vi "main.vi"() -> ()   [LabVIEW 2016]
uses:
  Classes/Controller/Motion/A3200 Folder/A3200.lvclass
  D:/Gantry_General/Classes/Controller/Motion/Motion Folder/Motion.lvclass
  Classes/Controller/I-O/NI-DAQ Folder/NI-DAQ.lvclass
  Classes/Controller/Dispenser/Ultimus V2 Folder/Ultimus V2.lvclass
  Classes/Controller/Motion/Motion Folder/Motion.lvclass
panel:
  in  "go patten":bool
  in  "tool go":bool
  in  "Tab Control":T1(tab)=enum."motion"
  in  "motion":T2={"XYZU "=[], "XY speed"=18.0, "Z speed"=3.0, "U speed"=0.0}
  in  "XY go":bool
  in  "Z move to zero":bool
  out "gule distances":dbl[](array[numeric])=[-11.318999999999999]
  out "needle XYZTheta In":dbl[](array[numeric])=[725.0, 1030.0, 65.0, 0.0]
  in  "needle xy":dbl[](array[numeric])=[725.0, 1030.0]
  in  "move to needle position":bool
  in  "XY":dbl[](array[numeric])=[650.0, 1030.0]
  in  "Z Go":bool
  in  "Position":dbl=65.0 format="%#_13g"
  out "j sum":dbl[](array[numeric])=[942.6350010227258, 1089.1437265164827, 59.912692205840095, 6.588294085890035e-07]
  in  "joystick and camera":bool
  in  "Camera to assembly center":bool
  out "Camera sensor center":dbl[](array[numeric])=[1019.0492232692902, 801.895067350325]
  in  "Camera to sensor center":bool
  out "sensor angle":dbl=0.7658874276042356
  in  "get sensor center":bool
  in  "get assembly center":bool
  out "Syringe offset":dbl[](array[numeric])=[-219.26459939197957, -70.034558660843, 5.209704694303774, -1.287105754835295e-06]
  out "Camera assembly center":dbl[](array[numeric])=[988.450879710852, 1092.9842118849685]
  in  "Syringe to assembly center":bool
  out "Syringe CAD center":dbl[](array[numeric])=[769.1862803188724, 1022.9496532241255]
  out "assembly angle":dbl=0.807055390089498
  in  "get Syringe offset":bool
  in  "dispense":T3={"Vacuum Setting (0000)"=200, "Pressure"=30, "on delay (ms)"=300.0, "off delay (ms) "=600.0} {"Vacuum Setting (0000)" min=0 max=1000 step=1 format="%04.0f"}
  in  "new/data":bool
  in  "dispense change status":bool
  in  "IO":cluster{"Output num":dbl[], "Output ":bool[]}={"Output num"=[11.0], "Output "=[FALSE]}
  in  "IO on /off":bool
  in  "Indices":i32[](array[numeric])=[11]
  in  "Values":bool[](array[boolean])=[TRUE]
  out "subarray":bool[](array[boolean])
  in  "z offset":T4={"Syringe Z0"=65.0, "assembly thickness"=1.219, "tool height"=9.5, "Gule thickness "=0.1, "Pick Up Tool Z height"=63.0289, "assembly Z offset"=-4.86, "gule distances"=0.6, "Syringe Z height abs"=53.681, "assembly Z height abs"=56.6499, "Syringe Z height rel"=-11.318999999999999, "assembly Z height rel"=-1.5190000000000001, "component  thickness"=0.2}
  in  "file path (dialog if empty)":path=path "D:/Gantry_General/Main/ms_kao/data/CAD patten/CAD PCB full 0.8 P30 20210608/CAD PCB full 0.8 P30 20210608.txt"
  in  "stop":bool
  in  "go CAD":bool
  in  "XY new Speed":dbl=25.0
  # "點膠速度"
  # "設定新速度"
  # "使用新/資料速度"
  # "間距70 mm"
  # "(1050, 865)\n(1050, 935)\n(1050,1005)"
  # "(910, 865)\n(910, 935)\n(910,1005)"
  # "(980, 865)\n(980, 935)\n(980,1005)"
  # "(840, 865)\n(840, 935)\n(840,1005)"
  # "0.6"
  # "PCB 1.2"
  # "sensor 0.32 ,0.2 ,0.1 mm"
  # "9.5mm"
  # "PCB 1.21"
  # "Gule 0.1mm"
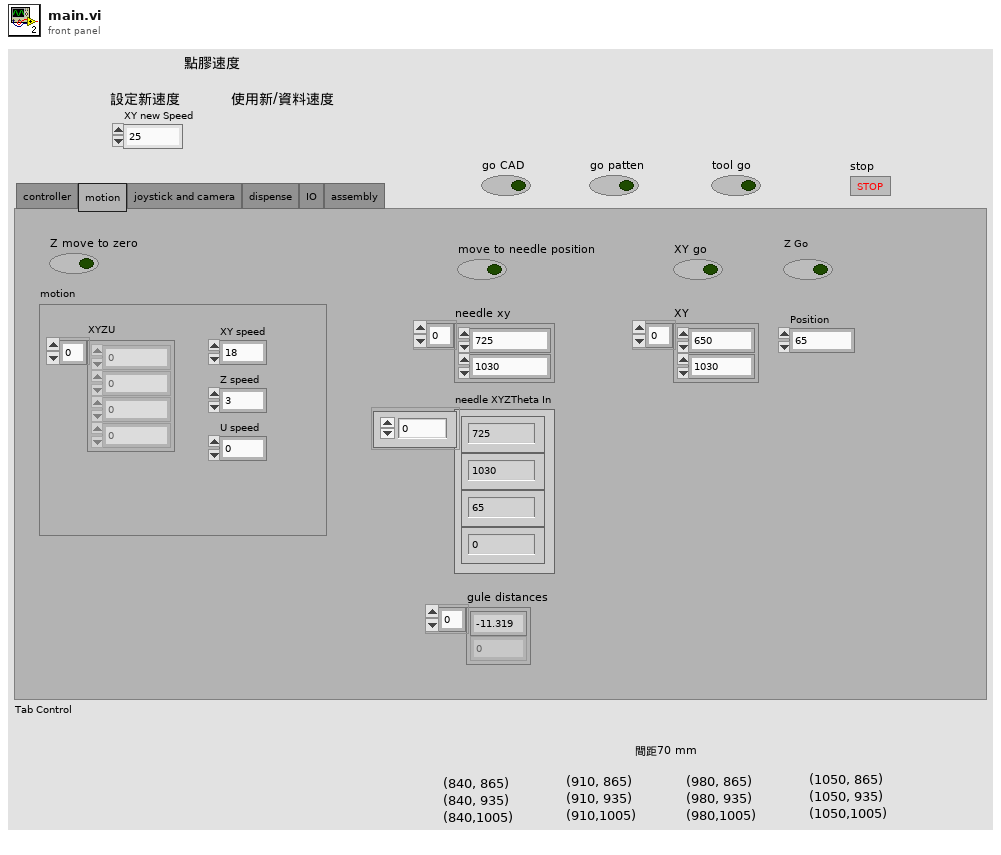
[diagram p1: front panel]
types:
  T1 = enum32{"controller", "motion", "joystick and camera", "dispense", "IO", "assembly"}
  T2 = cluster{"XYZU ":dbl[], "XY speed":dbl, "Z speed":dbl, "U speed":dbl}
  T3 = cluster{"Vacuum Setting (0000)":i64, "Pressure":i16, "on delay (ms)":dbl, "off delay (ms) ":dbl}
  T4 = cluster{"Syringe Z0":dbl, "assembly thickness":dbl, "tool height":dbl, "Gule thickness ":dbl, "Pick Up Tool Z height":dbl, "assembly Z offset":dbl, "gule distances":dbl, "Syringe Z height abs":dbl, "assembly Z height abs":dbl, "Syringe Z height rel":dbl, "assembly Z height rel":dbl, "component  thickness":dbl}
  T5 = cluster{"controller":cluster{"A3200.lvclass":refnum<class "A3200.lvclass">, "Ultimus V2.lvclass":refnum<class "Ultimus V2.lvclass">, "NI-DAQ.lvclass":refnum<class "NI-DAQ.lvclass">, "Motion.lvclass":refnum<class "Motion.lvclass">, "I-O.lvclass":refnum<class "I-O.lvclass">, "Dispenser.lvclass":refnum<class "Dispenser.lvclass">}, "folder and file name":cluster{"Path":path, "folder name":string, "file name":string, "extension":string, "add time string":bool}, "IO":cluster{"Output num":dbl[], "Output ":bool[]}, "motion":cluster{"XYZU ":dbl[], "XY speed":dbl, "Z speed":dbl, "U speed":dbl}, "dispense":cluster{"Vacuum Setting (0000)":i64, "Pressure":i16, "on delay (ms)":dbl, "off delay (ms) ":dbl}, "draw point Cluster":cluster{"dispense":bool, "Line/circle":bool, "ccw/cw":bool, "pressure":dbl, "speed":dbl, "start":dbl[], "end":dbl[], "center":dbl[], "Vacuum":dbl}}
  T6 = cluster{"A3200.lvclass":refnum<class "A3200.lvclass">, "Ultimus V2.lvclass":refnum<class "Ultimus V2.lvclass">, "NI-DAQ.lvclass":refnum<class "NI-DAQ.lvclass">, "Motion.lvclass":refnum<class "Motion.lvclass">, "I-O.lvclass":refnum<class "I-O.lvclass">, "Dispenser.lvclass":refnum<class "Dispenser.lvclass">}
  T7 = cluster{"Syringe offset":dbl[], "Camera assembly center":dbl[], "assembly angle":dbl, "Syringe CAD center":dbl[], "Camera sensor center":dbl[], "sensor angle":dbl}
  T8 = cluster{"dispense":bool, "Line/circle":bool, "ccw/cw":bool, "pressure":dbl, "speed":dbl, "start":dbl[], "end":dbl[], "center":dbl[], "Vacuum":dbl}[]
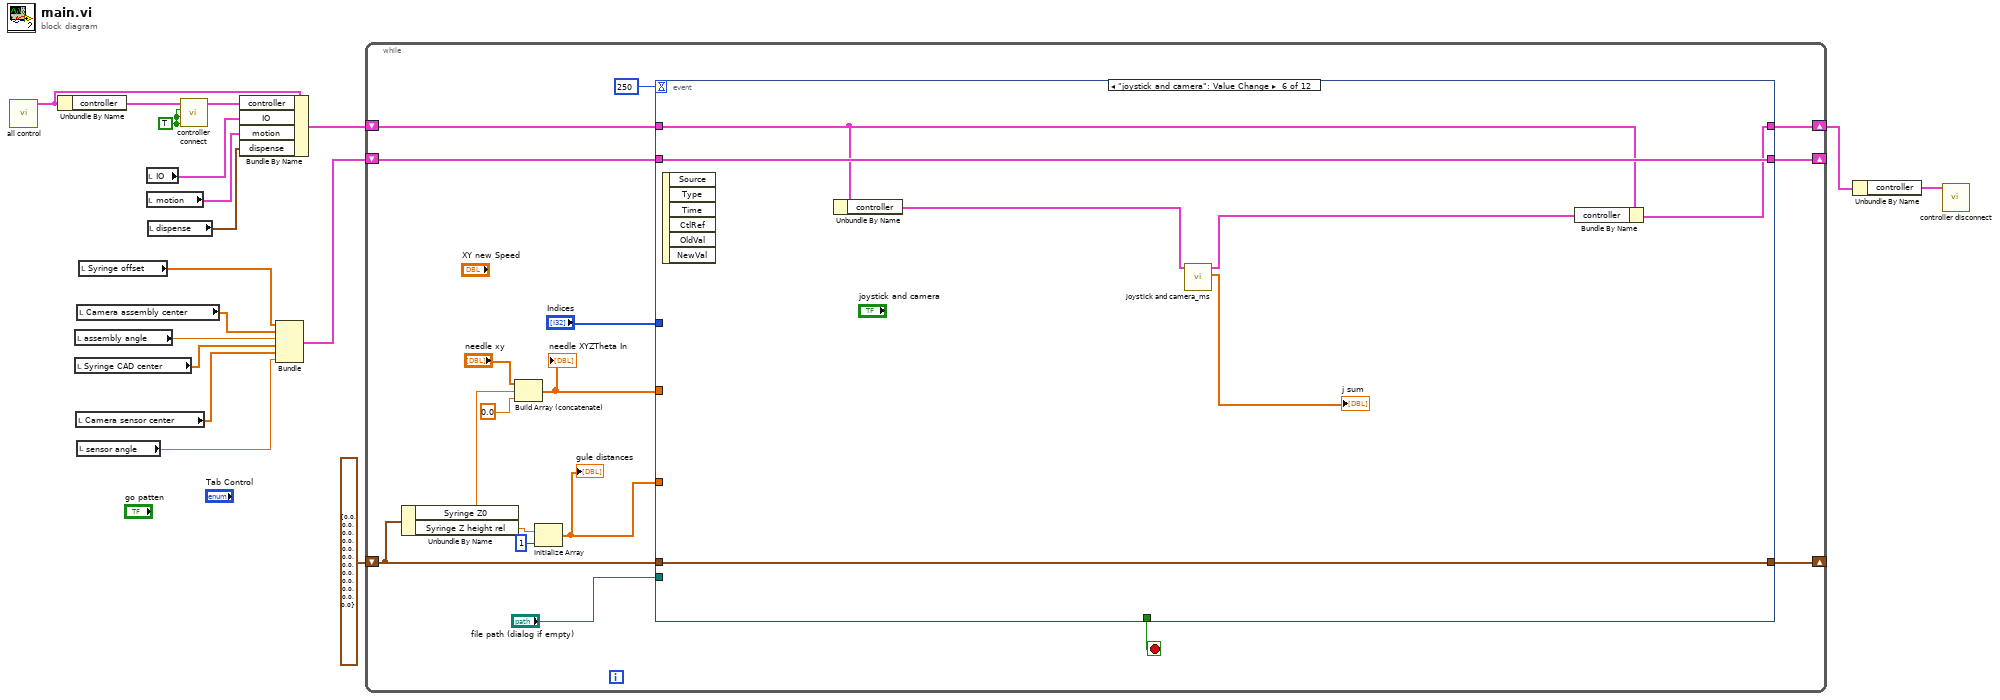
[diagram p0: block diagram]
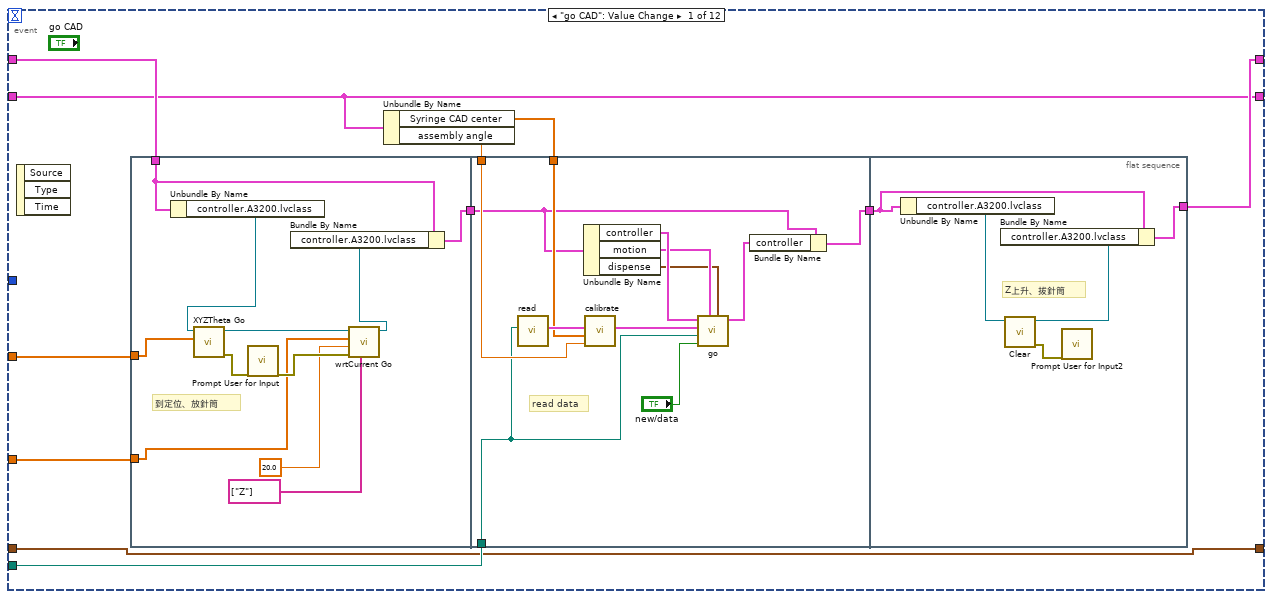
[diagram p2: hidden frame]
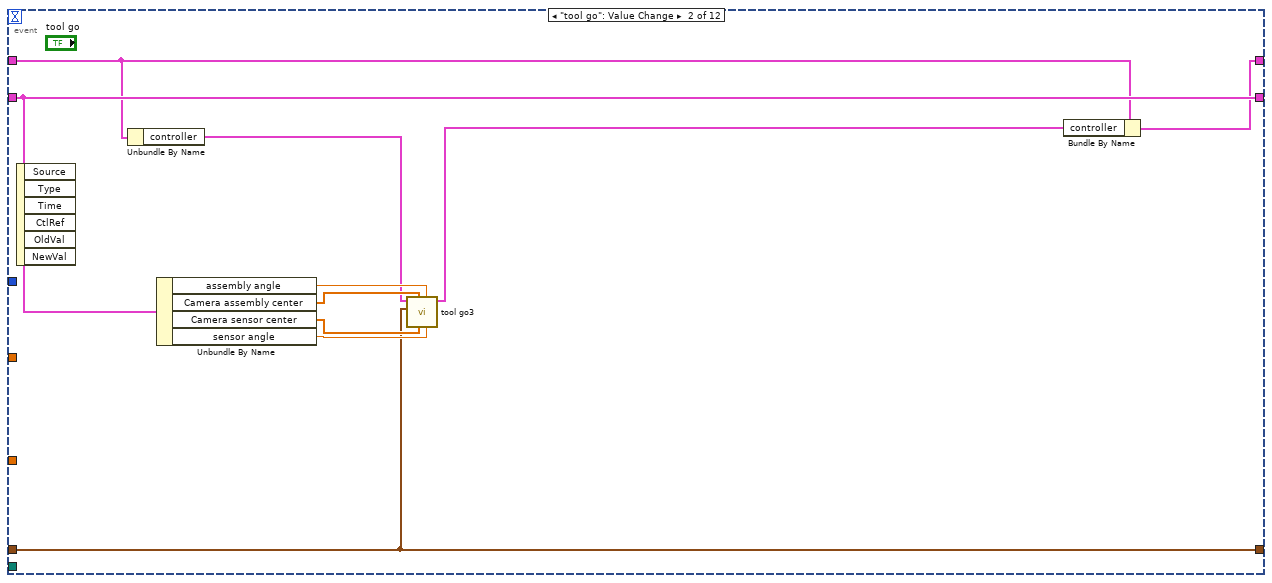
[diagram p3: hidden frame]
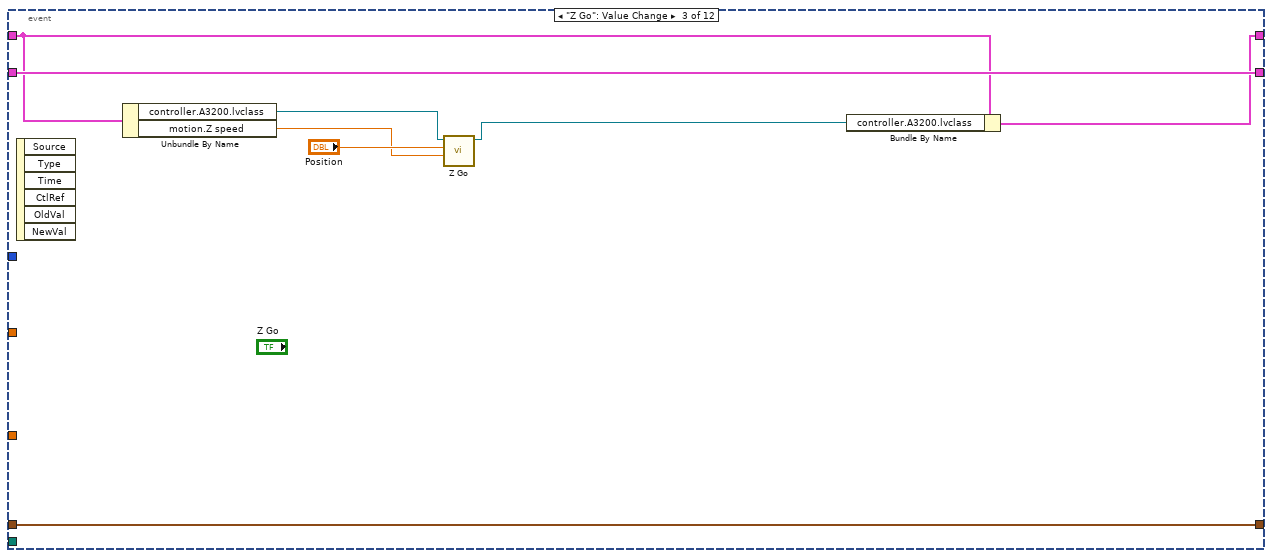
[diagram p4: hidden frame]
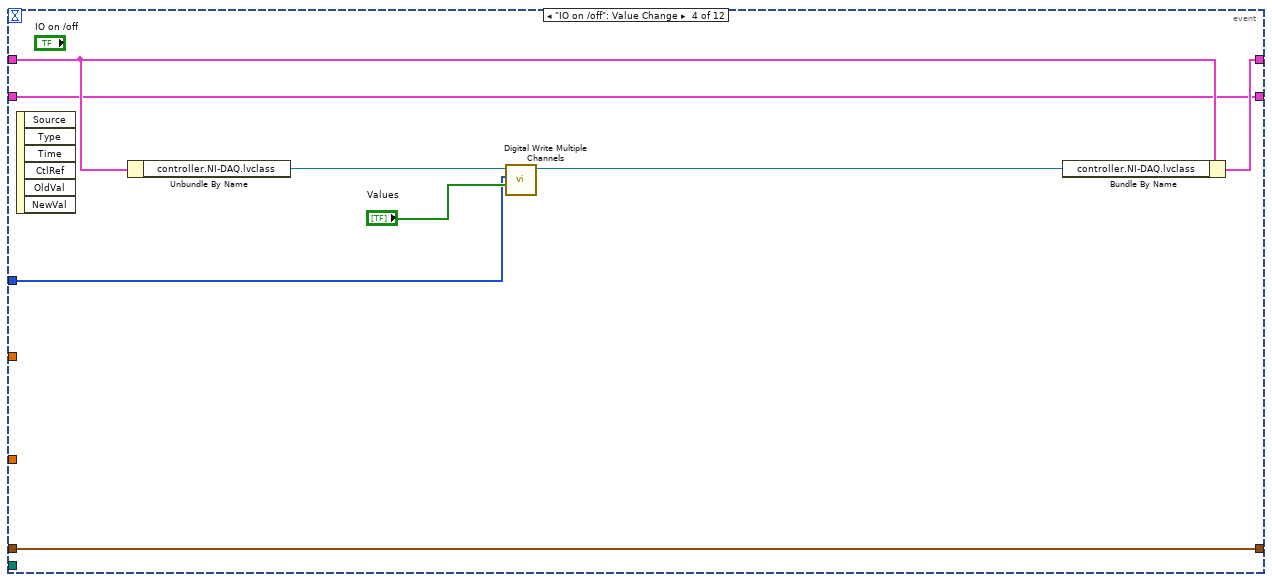
[diagram p5: hidden frame]
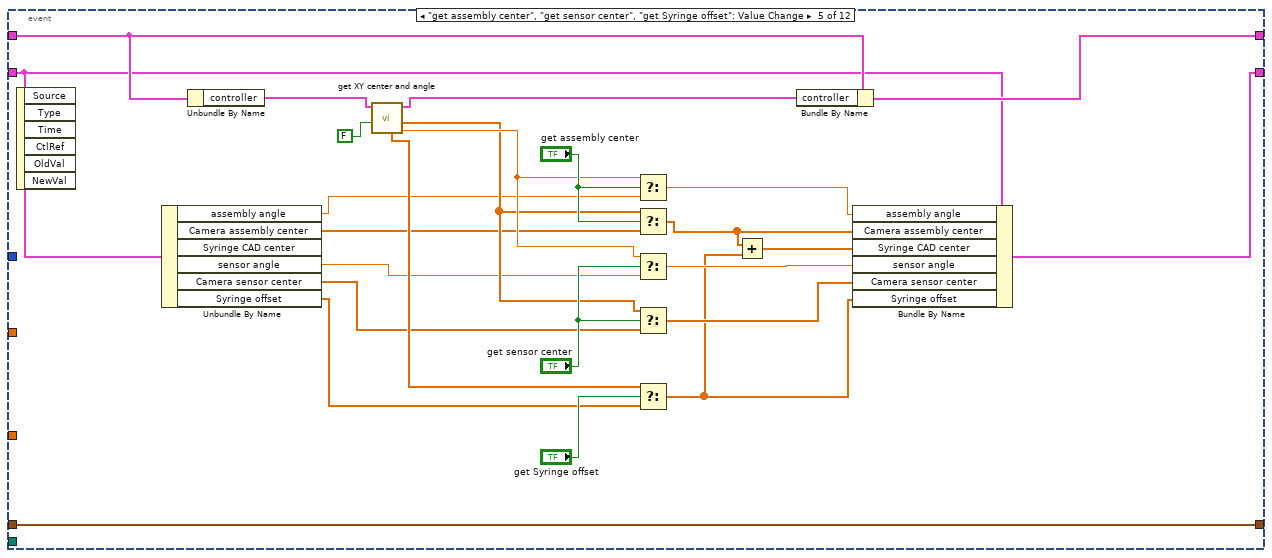
[diagram p6: hidden frame]
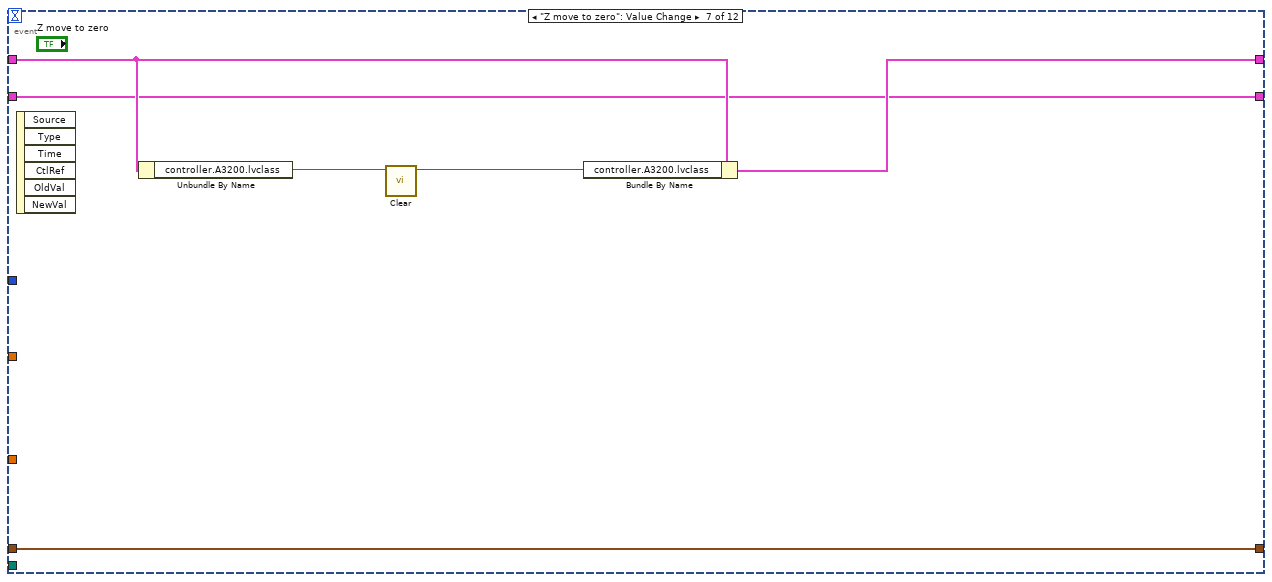
[diagram p7: hidden frame]
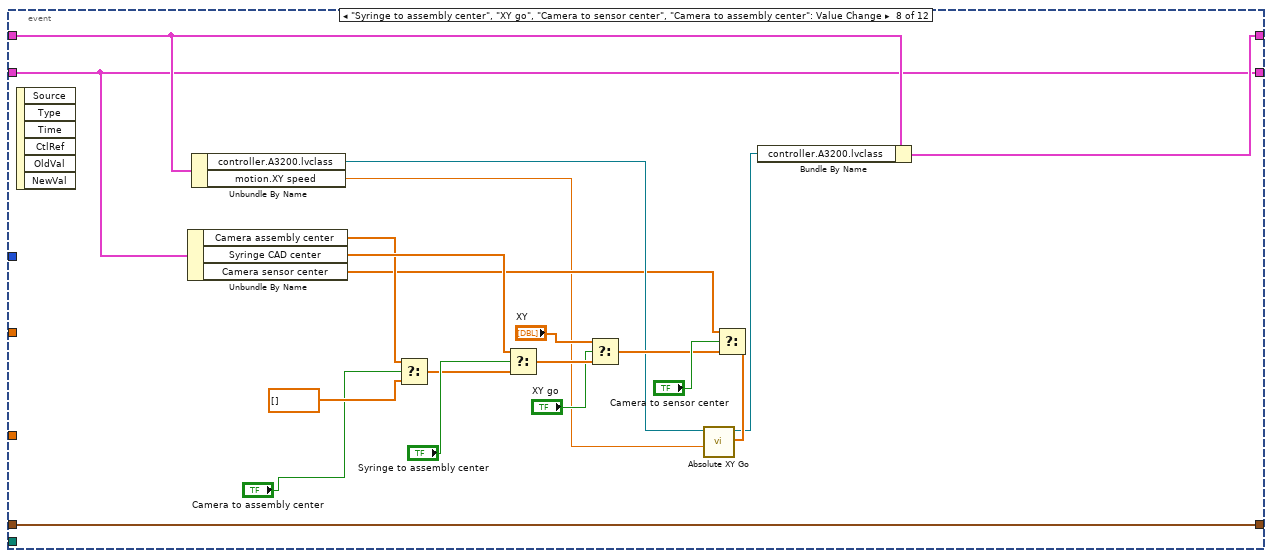
[diagram p8: hidden frame]
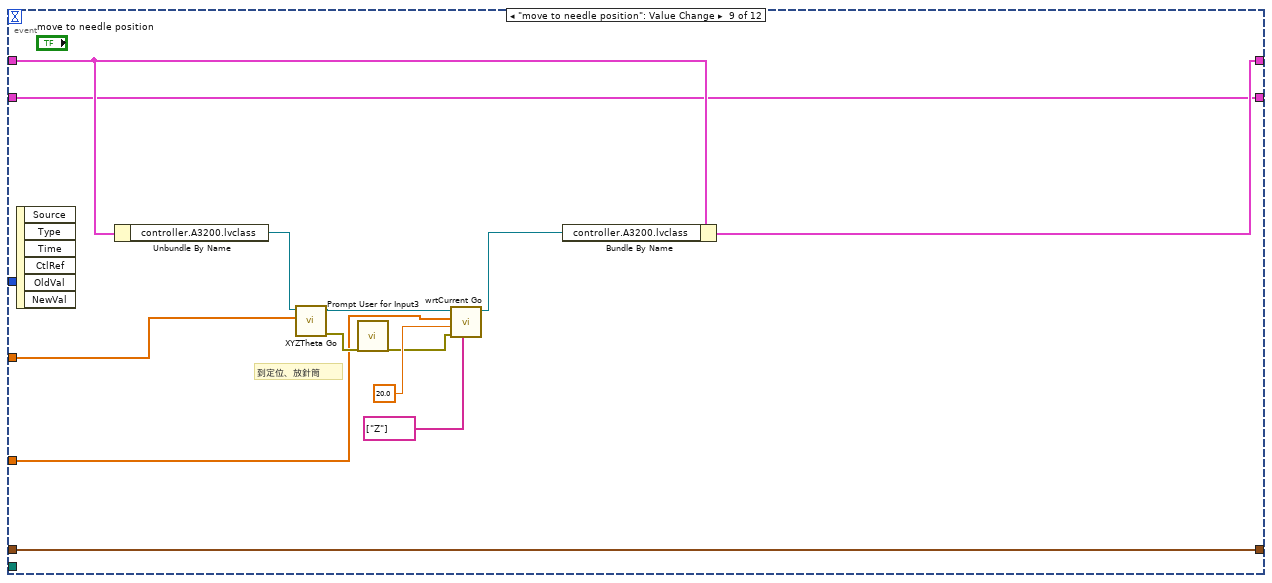
[diagram p9: hidden frame]
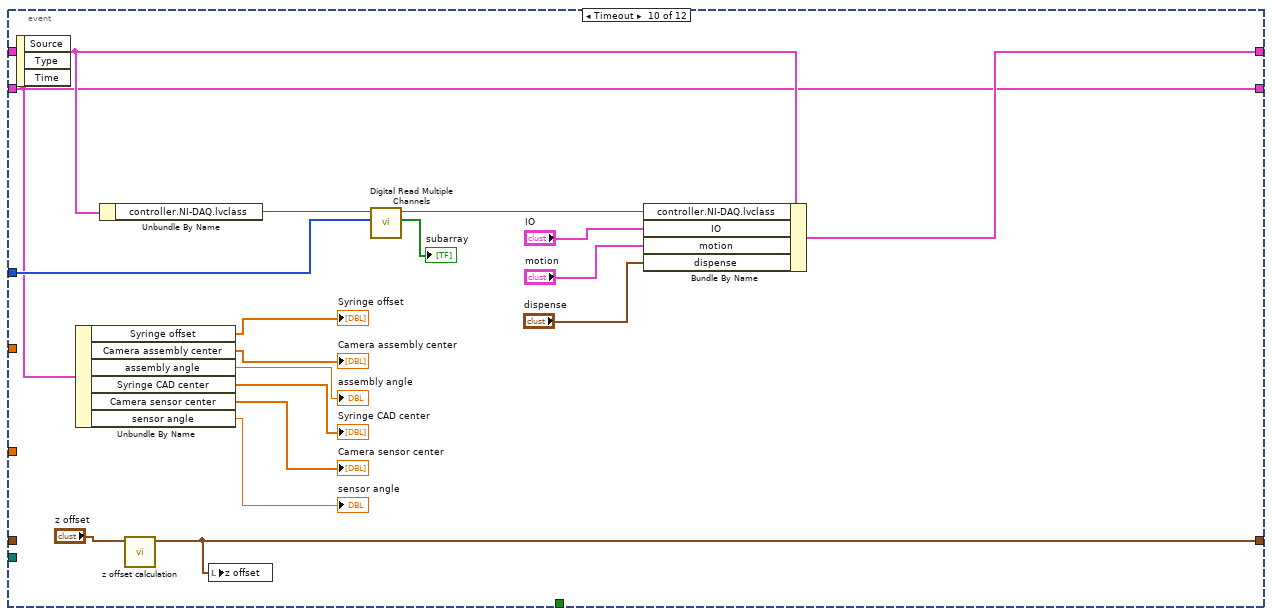
[diagram p10: hidden frame]
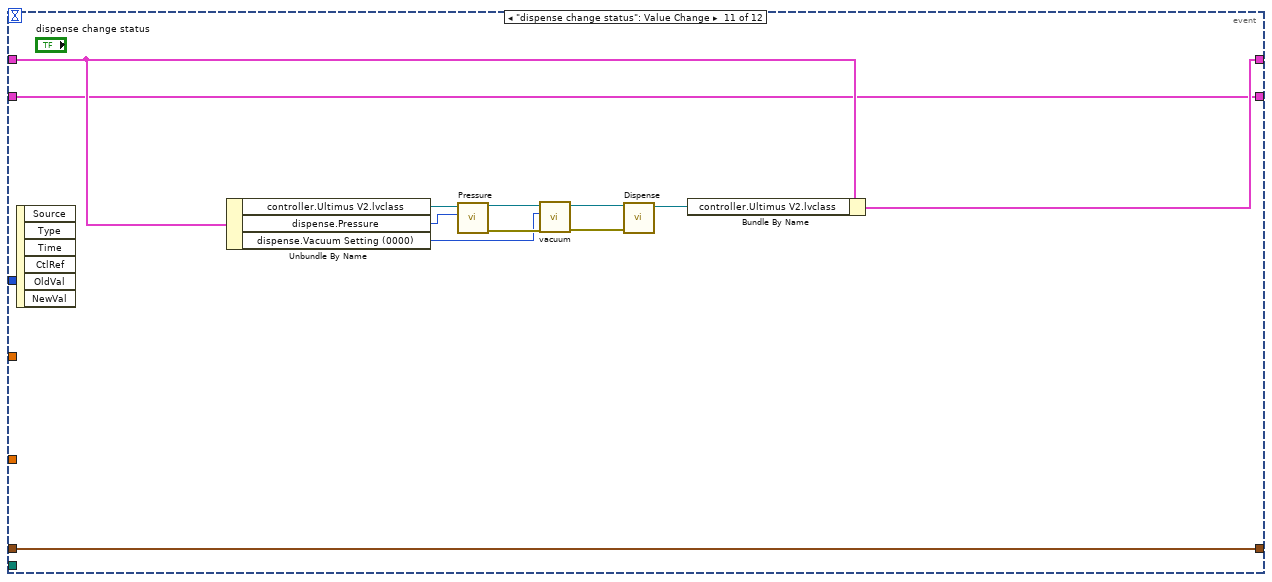
[diagram p11: hidden frame]
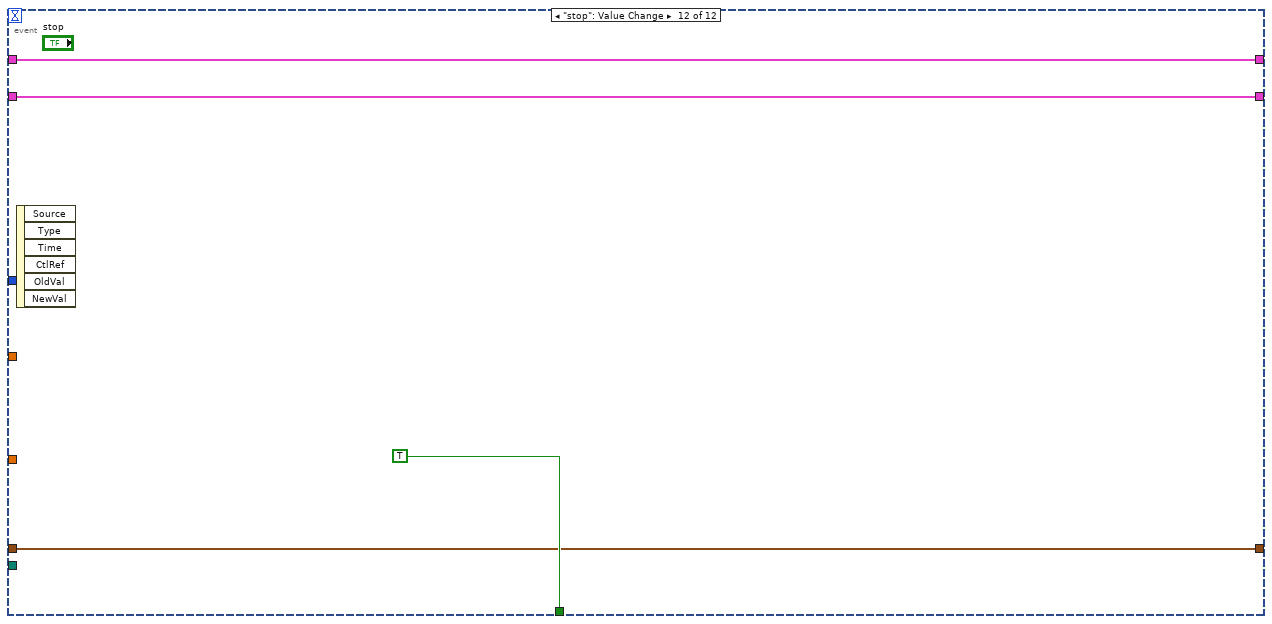
[diagram p12: hidden frame]
diagram:
  w18 = TRUE ("IO on")
  n1 = call "all control.vi"() -> ("output cluster"=w15:T5)  [unwired: 11 in]
  n2 = Unbundle By Name(w15) -> ("controller"=w17:T6)
  n3 = local read "assembly angle"() -> (w6:dbl)
  n4 = local read "Syringe CAD center"() -> (w5:dbl[])
  n5 = local read "Camera sensor center"() -> (w4:dbl[])
  n6 = local read "Camera assembly center"() -> (w7:dbl[])
  n7 = local read "sensor angle"() -> (w3:dbl)
  n8 = local read "Syringe offset"() -> (w8:dbl[])
  n9 = local read "IO"() -> (w9:cluster{"Output num":dbl[], "Output ":bool[]})
  n10 = local read "motion"() -> (w10:T2)
  n11 = local read "dispense"() -> (w11:T3)
  n12 = call "controller connect.vi"("IO on"=w18, "dispencer on"=w18, "motion on"=w18, "controller in"=w17) -> ("controller out"=w16:T6)  [unwired: 7 in]
  n13 = Bundle By Name(cluster=w15, "controller"=w16, "IO"=w9, "motion"=w10, "dispense"=w11) -> (w14:T5)
  n14 = Bundle("Syringe offset"=w8, "Camera assembly center"=w7, "assembly angle"=w6, "Syringe CAD center"=w5, "Camera sensor center"=w4, "sensor angle"=w3) -> (w2:T7)  [unwired: 1 in]
  n15 = while {
    shift-right: [w27] -> w13
    shift-left: w14 -> [w28]
    shift-right: [w25] -> _
    shift-left: w2 -> [w26]
    shift-right: [w24] -> _
    shift-left: T4 {"Syringe Z0"=0.0, "assembly thickness"=0.0, "tool height"=0.0, "Gule thickness "=0.0, "Pick Up Tool Z height"=0.0, "assembly Z offset"=0.0, "gule distances"=0.0, "Syringe Z height abs"=0.0, "assembly Z height abs"=0.0, "Syringe Z height rel"=0.0, "assembly Z height rel"=0.0, "component  thickness"=0.0} ("z offset out") -> [w23]
    stop <- w35 stop-if-true
    n16 = Unbundle By Name(w23) -> ("Syringe Z0"=w22:dbl, "Syringe Z height rel"=w21:dbl)
    n17 = Build Array (concatenate)("needle xy", w22, 0.0 ("element")) -> (w34:dbl[])
    "needle XYZTheta In" <- w34
    n18 = Initialize Array(w21, 1 ("dimension size")) -> (w20:dbl[])
    "gule distances" <- w20
    n19 = event shown="[5] \"joystick and camera\": Value Change" {
      selector: _ -> [_ _ _ _ _ _ _ _ _ _ _ _]
      dyn-events: _ -> [_ _ _ _ _ _ _ _ _ _ _ _]
      timeout: 250 -> [_ _ _ _ _ _ _ _ _ _ _ _]
      tunnel: [_ _ _ _ _ _ _ _ _ _ _ TRUE] -> w35
      tunnel: w34 -> [w45 _ _ _ _ _ _ _ w168 _ _ _]
      tunnel: w20 -> [w46 _ _ _ _ _ _ _ w159 _ _ _]
      tunnel: "Indices" -> [_ _ _ w99 _ _ _ _ _ w188 _ _]
      tunnel: "file path (dialog if empty)" -> [w37 _ _ _ _ _ _ _ _ _ _ _]
      tunnel: w28 -> [w44 w77 w87 w98 w118 w128 w137 w147 w166 w185 w201 w204]
      tunnel: [w41 w78 w86 w97 w117 w129 w138 w148 w165 w184 w200 w204] -> w27
      tunnel: w26 -> [w40 w84 w92 w94 w111 w132 w134 w144 w163 w180 w196 w203]
      tunnel: [w40 w84 w92 w94 w110 w132 w134 w144 w163 w180 w196 w203] -> w25
      tunnel: w23 -> [w36 w75 w91 w93 w101 w126 w133 w139 w160 _ w190 w202]
      tunnel: [w36 w75 w91 w93 w101 w126 w133 w139 w160 w172 w190 w202] -> w24
      event "go CAD": Value Change {
        n20 = event-data() -> ()  [unwired: 1 in, 3 out]
        n21 = flat-sequence {
          tunnel: w46 -> [w52]
          tunnel: w45 -> [w51]
          tunnel: w44 -> [w49]
          tunnel: [w48] -> w43
          tunnel: w43 -> [w60]
          tunnel: [w59] -> w42
          tunnel: w39 -> [w63]
          tunnel: w38 -> [w62]
          tunnel: w37 -> [w61]
          tunnel: w42 -> [w71]
          tunnel: [w70] -> w41
          frame #0 {
            # "到定位、放針筒"
            n22 = Unbundle By Name(w49) -> ("controller.A3200.lvclass"=w50:refnum<class "A3200.lvclass">)
            n23 = call "XYZTheta Go.vi"("XYZTheta In"=w51, "Motion in"=w50) -> ("error out"=w53:errorcluster, "Motion out"=w56:refnum<class "A3200.lvclass">)  [unwired: 7 in, 1 out]
            n24 = call "Prompt User for Input"("error in (no error)"=w53) -> ("error out"=w57:errorcluster)  [unwired: 17 in, 1 out]
            n25 = call-dynamic "wrtCurrent Go.vi"("axis names"=string[] ["Z"], "error in (no error)"=w57, "Speed"=20.0, "distances"=w52, "A3200 in"=w56) -> ("A3200 out"=w47:refnum<class "A3200.lvclass">)  [unwired: 5 in, 1 out]
            n26 = Bundle By Name(cluster=w49, "controller.A3200.lvclass"=w47) -> (w48:T5)
          }
          frame #1 {
            # "read data"
            n27 = call "read.vi"("file path (dialog if empty)"=w61) -> ("Array"=w69:T8)  [unwired: 9 in]
            n28 = Unbundle By Name(w60) -> ("controller"=w68:T6, "motion"=w67:T2, "dispense"=w66:T3)
            n29 = call "calibrate.vi"("angle"=w62, "CAD center"=w63, "Array 3"=w69) -> ("Array 2"=w65:T8)  [unwired: 8 in]
            n30 = call "go.vi"("dispense"=w66, "motion"=w67, "use new/data"="new/data", "file path (dialog if empty)"=w61, "cluster Array input"=w65, "controller in"=w68) -> ("controller out"=w58:T6)  [unwired: 5 in]
            n31 = Bundle By Name(cluster=w60, "controller"=w58) -> (w59:T5)
          }
          frame #2 {
            # "Z上升、拔針筒"
            n32 = Unbundle By Name(w71) -> ("controller.A3200.lvclass"=w73:refnum<class "A3200.lvclass">)
            n33 = call "Clear.vi"("Motion in"=w73) -> ("error out"=w74:errorcluster, "Motion out"=w72:refnum<class "A3200.lvclass">)  [unwired: 9 in]
            n34 = Bundle By Name(cluster=w71, "controller.A3200.lvclass"=w72) -> (w70:T5)
            n35 = call "Prompt User for Input2"("error in (no error)"=w74) -> ()  [unwired: 17 in, 2 out]
          }
        }
        n36 = Unbundle By Name(w40) -> ("Syringe CAD center"=w39:dbl[], "assembly angle"=w38:dbl)
      }
      event "tool go": Value Change {
        n37 = event-data() -> ()  [unwired: 1 in, 6 out]
        n38 = Unbundle By Name(w77) -> ("controller"=w79:T6)
        n39 = Unbundle By Name(w84) -> ("assembly angle"=w82:dbl, "Camera assembly center"=w83:dbl[], "Camera sensor center"=w81:dbl[], "sensor angle"=w80:dbl)
        n40 = call "tool go3.vi"("sensor angle"=w80, "assembly angle"=w82, "sensor center"=w81, "assembly center"=w83, "z offset"=w75, "controller in"=w79) -> ("controller out"=w76:T6)  [unwired: 4 in, 1 out]
        n41 = Bundle By Name(cluster=w77, "controller"=w76) -> (w78:T5)
      }
      event "Z Go": Value Change {
        n42 = event-data() -> ()  [unwired: 1 in, 6 out]
        n43 = Unbundle By Name(w87) -> ("controller.A3200.lvclass"=w88:refnum<class "A3200.lvclass">, "motion.Z speed"=w89:dbl)
        n44 = call-dynamic "Z Go.vi"("Speed"=w89, "Position"="Position", "Gantry in"=w88) -> ("Gantry out"=w85:refnum<class "A3200.lvclass">)  [unwired: 7 in, 1 out]
        n45 = Bundle By Name(cluster=w87, "controller.A3200.lvclass"=w85) -> (w86:T5)
      }
      event "IO on /off": Value Change {
        n46 = event-data() -> ()  [unwired: 1 in, 6 out]
        n47 = Unbundle By Name(w98) -> ("controller.NI-DAQ.lvclass"=w95:refnum<class "NI-DAQ.lvclass">)
        n48 = call-dynamic "Digital Write Multiple Channels.vi"("Values"="Values", "Indices"=w99, "NI-DAQ in"=w95) -> ("NI-DAQ out"=w96:refnum<class "NI-DAQ.lvclass">)  [unwired: 7 in, 1 out]
        n49 = Bundle By Name(cluster=w98, "controller.NI-DAQ.lvclass"=w96) -> (w97:T5)
      }
      event "get assembly center", "get sensor center", "get Syringe offset": Value Change {
        n50 = event-data() -> ()  [unwired: 1 in, 6 out]
        n51 = Unbundle By Name(w111) -> ("assembly angle"=w116:dbl, "Camera assembly center"=w115:dbl[], "sensor angle"=w114:dbl, "Camera sensor center"=w113:dbl[], "Syringe offset"=w112:dbl[])  [unwired: 1 out]
        n52 = Unbundle By Name(w118) -> ("controller"=w103:T6)
        n53 = call "get XY center and angle.vi"("output P1 XY"=FALSE, "controller in"=w103) -> ("XY theta out"=w123:dbl, "XY center out"=w122:dbl[], "controller out"=w102:T6, "offset P1-P2"=w120:dbl[])  [unwired: 6 in]
        n54 = Select(t=w123, s="get assembly center", f=w116) -> (s? t:f=w107:dbl)
        n55 = Select(t=w122, s="get assembly center", f=w115) -> (s? t:f=w105:dbl[])
        n56 = Select(t=w123, s="get sensor center", f=w114) -> (s? t:f=w108:dbl)
        n57 = Select(t=w122, s="get sensor center", f=w113) -> (s? t:f=w109:dbl[])
        n58 = Select(t=w120, s="get Syringe offset", f=w112) -> (s? t:f=w104:dbl[])
        n59 = Add(x=w105, y=w104) -> (x+y=w106:dbl[])
        n60 = Bundle By Name(cluster=w118, "controller"=w102) -> (w117:T5)
        n61 = Bundle By Name(cluster=w111, "assembly angle"=w107, "Camera assembly center"=w105, "Syringe CAD center"=w106, "sensor angle"=w108, "Camera sensor center"=w109, "Syringe offset"=w104) -> (w110:T7)
      }
      event "joystick and camera": Value Change {
        n62 = event-data() -> ()  [unwired: 1 in, 6 out]
        n63 = Unbundle By Name(w128) -> ("controller"=w130:T6)
        n64 = call "joystick and camera_ms.vi"("controller in"=w130) -> ("Gantry"=→"j sum":dbl[], "controller out"=w131:T6)  [unwired: 9 in]
        n65 = Bundle By Name(cluster=w128, "controller"=w131) -> (w129:T5)
      }
      event "Z move to zero": Value Change {
        n66 = event-data() -> ()  [unwired: 1 in, 6 out]
        n67 = Unbundle By Name(w137) -> ("controller.A3200.lvclass"=w136:refnum<class "A3200.lvclass">)
        n68 = call "Clear.vi"("Motion in"=w136) -> ("Motion out"=w135:refnum<class "A3200.lvclass">)  [unwired: 9 in, 1 out]
        n69 = Bundle By Name(cluster=w137, "controller.A3200.lvclass"=w135) -> (w138:T5)
      }
      event "Syringe to assembly center", "XY go", "Camera to sensor center", "Camera to assembly center": Value Change {
        n70 = event-data() -> ()  [unwired: 1 in, 6 out]
        n71 = Unbundle By Name(w144) -> ("Camera assembly center"=w142:dbl[], "Syringe CAD center"=w143:dbl[], "Camera sensor center"=w141:dbl[])
        n72 = Unbundle By Name(w147) -> ("controller.A3200.lvclass"=w145:refnum<class "A3200.lvclass">, "motion.XY speed"=w140:dbl)
        n73 = Select(t=w142, s="Camera to assembly center", f=dbl[] []) -> (s? t:f=w150:dbl[])
        n74 = Select(t=w143, s="Syringe to assembly center", f=w150) -> (s? t:f=w157:dbl[])
        n75 = Select(t="XY", s="XY go", f=w157) -> (s? t:f=w153:dbl[])
        n76 = Select(t=w141, s="Camera to sensor center", f=w153) -> (s? t:f=w152:dbl[])
        n77 = call-dynamic "Absolute XY Go.vi"("Speed"=w140, "XY"=w152, "Gantry in"=w145) -> ("Gantry out"=w146:refnum<class "A3200.lvclass">)  [unwired: 7 in, 1 out]
        n78 = Bundle By Name(cluster=w147, "controller.A3200.lvclass"=w146) -> (w148:T5)
      }
      event "move to needle position": Value Change {
        # "到定位、放針筒"
        n79 = event-data() -> ()  [unwired: 1 in, 6 out]
        n80 = Unbundle By Name(w166) -> ("controller.A3200.lvclass"=w162:refnum<class "A3200.lvclass">)
        n81 = call "XYZTheta Go.vi"("XYZTheta In"=w168, "Motion in"=w162) -> ("error out"=w171:errorcluster, "Motion out"=w161:refnum<class "A3200.lvclass">)  [unwired: 7 in, 1 out]
        n82 = call "Prompt User for Input3"("error in (no error)"=w171) -> ("error out"=w169:errorcluster)  [unwired: 17 in, 1 out]
        n83 = call-dynamic "wrtCurrent Go.vi"("axis names"=string[] ["Z"], "error in (no error)"=w169, "Speed"=20.0, "distances"=w159, "A3200 in"=w161) -> ("A3200 out"=w164:refnum<class "A3200.lvclass">)  [unwired: 5 in, 1 out]
        n84 = Bundle By Name(cluster=w166, "controller.A3200.lvclass"=w164) -> (w165:T5)
      }
      event Timeout {
        n85 = event-data() -> ()  [unwired: 1 in, 3 out]
        n86 = Unbundle By Name(w180) -> ("Syringe offset"=→"Syringe offset":dbl[], "Camera assembly center"=→"Camera assembly center":dbl[], "assembly angle"=→"assembly angle":dbl, "Syringe CAD center"=→"Syringe CAD center":dbl[], "Camera sensor center"=→"Camera sensor center":dbl[], "sensor angle"=→"sensor angle":dbl)
        n87 = Unbundle By Name(w185) -> ("controller.NI-DAQ.lvclass"=w187:refnum<class "NI-DAQ.lvclass">)
        n88 = call "z offset calculation.vi"("z offset in"="z offset") -> ("z offset out"=w172:T4)  [unwired: 10 in]
        n89 = local write "z offset"(w172) -> ()
        n90 = call-dynamic "Digital Read Multiple Channels.vi"("Array"=w188, "NI-DAQ in"=w187) -> ("subarray"=→"subarray":bool[], "NI-DAQ out"=w186:refnum<class "NI-DAQ.lvclass">)  [unwired: 7 in, 1 out]
        n91 = Bundle By Name(cluster=w185, "controller.NI-DAQ.lvclass"=w186, "IO"="IO", "motion"="motion", "dispense"="dispense") -> (w184:T5)
      }
      event "dispense change status": Value Change {
        n92 = event-data() -> ()  [unwired: 1 in, 6 out]
        n93 = Unbundle By Name(w201) -> ("controller.Ultimus V2.lvclass"=w199:refnum<class "Ultimus V2.lvclass">, "dispense.Pressure"=w198:i16, "dispense.Vacuum Setting (0000)"=w191:i64)
        n94 = call-dynamic "Pressure.vi"("Pressure"=w198, "Ultimus V in"=w199) -> ("error out"=w192:errorcluster, "Ultimus V out"=w195:refnum<class "Ultimus V2.lvclass">)  [unwired: 8 in]
        n95 = call "vacuum.vi"("error in (no error)"=w192, "Vacuum Setting (0000)"=w191, "Ultimus V in"=w195) -> ("error out"=w193:errorcluster, "Ultimus V out"=w194:refnum<class "Ultimus V2.lvclass">)  [unwired: 7 in]
        n96 = call-dynamic "Dispense.vi"("error in (no error)"=w193, "Ultimus V in"=w194) -> ("Ultimus V out"=w197:refnum<class "Ultimus V2.lvclass">)  [unwired: 8 in, 1 out]
        n97 = Bundle By Name(cluster=w201, "controller.Ultimus V2.lvclass"=w197) -> (w200:T5)
      }
      event "stop": Value Change {
        n98 = event-data() -> ()  [unwired: 1 in, 6 out]
      }
    }
  }
  n99 = Unbundle By Name(w13) -> ("controller"=w12:T6)
  n100 = call "controller disconnect.vi"("controller 2"=w12) -> ()  [unwired: 11 in]
